vi "Get Bucket Policy.vi"(8 "error in (no error)":errorcluster, 11 "Bucket in":refnum<class "Bucket.lvclass">) -> (0 "error out":errorcluster, 2 "Policy":string, 3 "Bucket out":refnum<class "Bucket.lvclass">)   [LabVIEW 2015, in "NI_AWS_S3.lvlib" / "Bucket.lvclass"]
doc: "This implementation of the GET operation uses the policy subresource to return the policy of a specified bucket. To use this operation, you must have GetPolicy permissions on the specified bucket, and you must be the bucket owner.\n\nIf you don't have GetPolicy permissions, Amazon S3 returns a 403 Access Denied error. If you have the correct permissions, but you're not the bucket owner, Amazon S3 returns a 405 Method Not Allowed error. If the bucket does not have a policy, Amazon S3 returns a 404 Policy Not found error. There are restrictions about who can create bucket policies and which objects in a bucket they can apply to."
uses:
  Bucket.lvclass
  Core/HTTP Request/Region handling.ctl
  Core/HTTP Request/Name Value Pair.ctl
  Core/HTTP Request/Request Options.ctl
  Core/HTTP Request/URL formatting.ctl
  Bucket.lvclass/Bucket.ctl
  Read Name.vi
  Core/HTTP Request/HTTP Request.lvclass
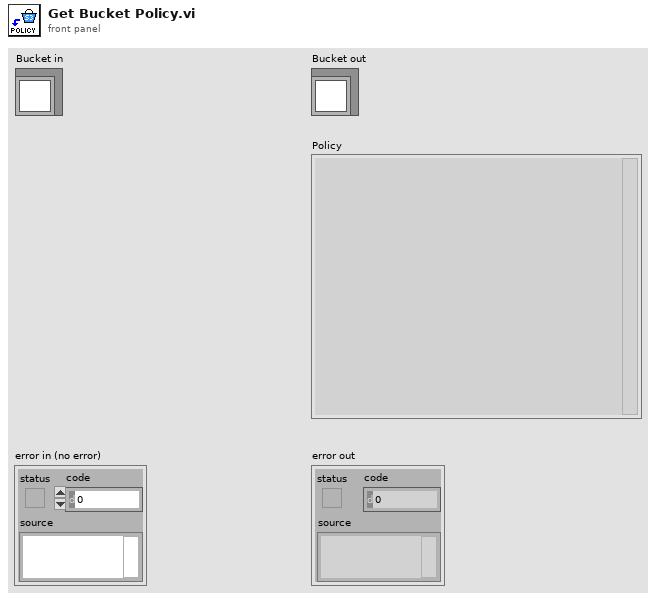
[diagram p1: front panel]
types:
  T1 = typedef "NI_AWS_Core.lvlib/HTTP Request.lvclass/Request Options.ctl" = cluster{"request headers":T2[], "request parameters":T2[], "request body":string, "region handling":T3, "URL formatting":T4}
  T2 = typedef "NI_AWS_Core.lvlib/HTTP Request.lvclass/Name Value Pair.ctl" = cluster{"name":string, "value":string}
  T3 = typedef "NI_AWS_Core.lvlib/HTTP Request.lvclass/Region handling.ctl" = enum16{"use region everywhere", "use region (authentication only)", "use region (URL only)", "ignore region everwhere"}
  T4 = typedef "NI_AWS_Core.lvlib/HTTP Request.lvclass/URL formatting.ctl" = enum16{"region-", "region."}
  T5 = typedef "NI_AWS_Core.lvlib/HTTP Request.lvclass/Response.ctl" = cluster{"Headers":string, "Body":string}
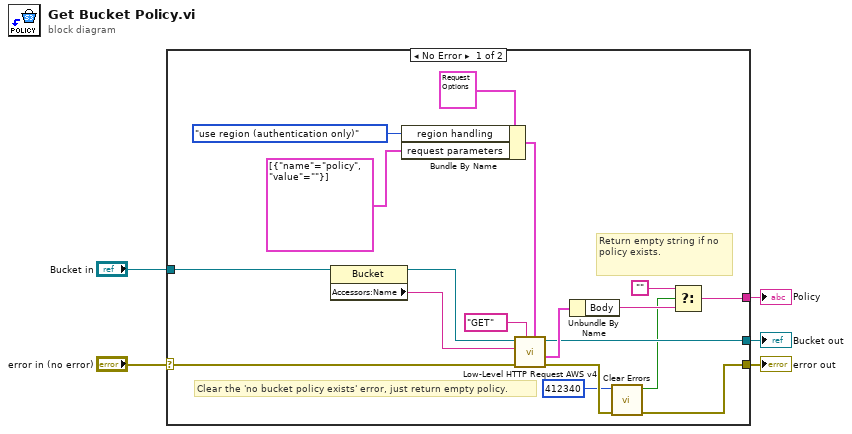
[diagram p0: block diagram]
diagram:
  n1 = case shown="No Error" "error in (no error)" {
    selector: "error in (no error)" -> [w19 w25]
    tunnel: "Bucket in" -> [w20 w24]
    tunnel: [w11 w25] -> w3
    tunnel: [w13 w24] -> w2
    tunnel: [w8 _] -> w1
    frame No Error {
      # "Return empty string if no policy exists."
      # "Clear the 'no bucket policy exists' error, just return empty policy."
      n2 = property class="Bucket"(reference=w20) -> (reference out=w14:refnum<class "Bucket.lvclass">, "Accessors:Name"=w23:string)  [unwired: 1 in, 1 out]
      n3 = Bundle By Name(cluster=T1 {"request headers"=[], "request parameters"=[], "request body"="", "region handling"=enum."use region everywhere", "URL formatting"=enum."region."} ("Request Options"), "region handling"=Region_handling."use region (authentication only)", "request parameters"=T2[] [{"name"="policy", "value"=""}]) -> (w15:T1)
      n4 = call "Low-Level HTTP Request AWS v4.vi"("Request Options"=w15, "HTTP-Verb"="GET", "error in (no error)"=w19, "URL Prefix"=w23, "AWS Core in"=w14) -> ("error out"=w12:errorcluster, "Response"=w17:T5, "AWS Core out"=w13:refnum<class "Bucket.lvclass">)  [unwired: 3 in, 1 out]
      n5 = Unbundle By Name(w17) -> ("Body"=w9:string)
      n6 = call <vilib>:"Clear Errors.vi"("error in (no error)"=w12, "specific error code to clear (0: all)"=412340) -> ("error out"=w11:errorcluster, "specific error cleared?"=w7:bool)  [unwired: 4 in]
      n7 = Select(t="", s=w7, f=w9) -> (s? t:f=w8:string)
    }
    frame Error {
    }
  }
  "error out" <- w3
  "Bucket out" <- w2
  "Policy" <- w1
